vi "return class name.vi"(11 "Class in":refnum<class>) -> (0 "error out":errorcluster, 3 "lowercase class name":string)   [LabVIEW 2020, in "Template.lvlib" / "Template.lvclass"]
doc: "Returns the class name from the parsed object"
uses:
  Template.lvclass
  <vilib>/regexp/Match Regular Expression.xnode
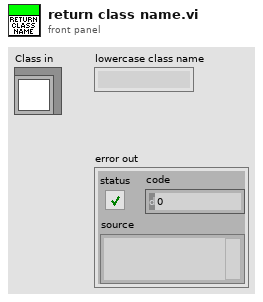
[diagram p1: front panel]
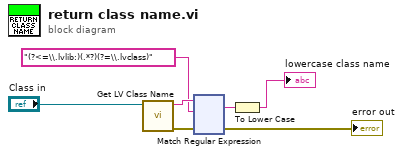
[diagram p0: block diagram]
diagram:
  n1 = call <vilib>:"Get LV Class Name.vi"("object"="Class in") -> ("error out"=w1:errorcluster, "class name"=w6:string)  [unwired: 9 in]
  n2 = xnode "Match Regular Expression"("input string"=w6, "regular expression"="(?<=\\.lvlib:)(.*?)(?=\\.lvclass)", "error in"=w1) -> ("whole match"=w5:string, "error out"=→"error out":errorcluster)  [unwired: 3 in, 3 out]
  n3 = To Lower Case(string=w5) -> (all lower case string=→"lowercase class name":string)
